vi "FormatData.vi"(10 "Array":string[](array[string])) -> (2 "data":string)   [LabVIEW 2016]
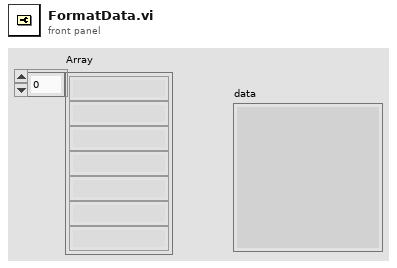
[diagram p1: front panel]
types:
  T1 = cluster{"index of element":i32, "String":string}[]
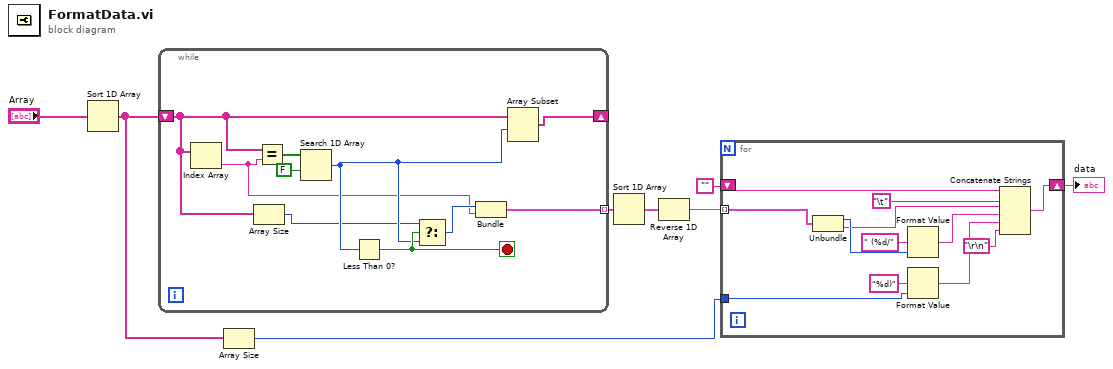
[diagram p0: block diagram]
diagram:
  n1 = Sort 1D Array(array="Array") -> (sorted array=w4:string[])
  n2 = while {
    shift-right: [w16] -> _
    shift-left: w4 -> [w12]
    tunnel: [w15] -> w7 mode=indexing
    stop <- w14 stop-if-true
    n3 = Index Array(array=w12) -> (element=w9:string)  [unwired: 1 in]
    n4 = Array Size(array=w12) -> (size(s)=w11:i32)
    n5 = Equal?(x=w12, y=w9) -> (x = y?=w18:bool[])
    n6 = Search 1D Array(1D array=w18, element=FALSE) -> (index of element=w13:i32)  [unwired: 1 in]
    n7 = Less Than 0?(x=w13) -> (x < 0?=w14:bool)
    n8 = Select(t=w11, s=w14, f=w13) -> (s? t:f=w10:i32)
    n9 = Bundle("index of element"=w10, "String"=w9) -> (w15:cluster{"index of element":i32, "String":string})  [unwired: 1 in]
    n10 = Array Subset(array=w12, index=w13) -> (w16:string[])  [unwired: 1 in]
  }
  n11 = Array Size(array=w4) -> (size(s)=w3:i32)
  n12 = Sort 1D Array(array=w7) -> (sorted array=w2:T1)
  n13 = Reverse 1D Array(array=w2) -> (reversed array=w1:T1)
  n14 = for {
    tunnel: w1 -> [w30] mode=indexing
    shift-right: [w27] -> w5
    shift-left: "" -> [w23]
    tunnel: w3 -> [w21]
    n15 = Unbundle(w30) -> ("index of element"=w20:i32, "String"=w19:string)
    n16 = Format Value(format string=" (%d/", value (0)=w20) -> (output string=w25:string)  [unwired: 1 in]
    n17 = Format Value(format string="%d)", value (0)=w21) -> (output string=w24:string)  [unwired: 1 in]
    n18 = Concatenate Strings(w23, "\t", w19, w25, w24, "\r\n") -> (w27:string)
  }
  "data" <- w5
